vi "Snap Camera Image.vi"(7 "Test Recipe in":refnum<class "Test Recipe.lvclass">, 10 "Camera":refnum<class "Camera.lvclass">, 11 "Path":path) -> (0 "error out":errorcluster, 2 "No Artifacts Found":bool, 3 "LEDs Found":u32)   [LabVIEW 2015, in "LED Board Test.lvclass"]
uses:
  LED Board Test.lvclass
  Classes/Instruments/Camera/Camera/Class/Camera.lvclass
  Classes/Test Recipe/Class/Test Recipe.lvclass
  Classes/Instruments/Camera/Camera/Vision Algorithm/Count LEDS on Image/Count LEDs on Image.lvclass
  Classes/Instruments/Camera/Camera/Vision Algorithm/Find Color Artifacts/Find Color Artifacts.lvclass
  Classes/Instruments/Camera/Camera/Vision Algorithm/Find Color Artifacts/Find Color Artifacts.lvclass/Find Color Artifacts.ctl
  Classes/Instruments/Camera/Camera/Vision Algorithm/Count LEDS on Image/Count LEDs on Image.lvclass/Count LEDs on Image.ctl
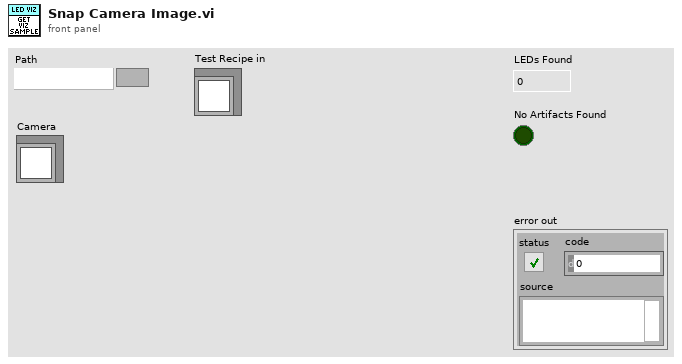
[diagram p1: front panel]
types:
  T1 = cluster{"Red Range":cluster{"Lower value":i32, "Upper value":i32}, "Green Range":cluster{"Lower value":i32, "Upper value":i32}, "Blue Range":cluster{"Lower value":i32, "Upper value":i32}}
  T2 = typedef "IMAQ Rectangle" = cluster{"Left":i32, "Top":i32, "Right":i32, "Bottom":i32, "Rotation":dbl}
  T3 = cluster{"Threshold":u32, "Min Size":u32, "Max Size":u32, "Use Max Size":bool}
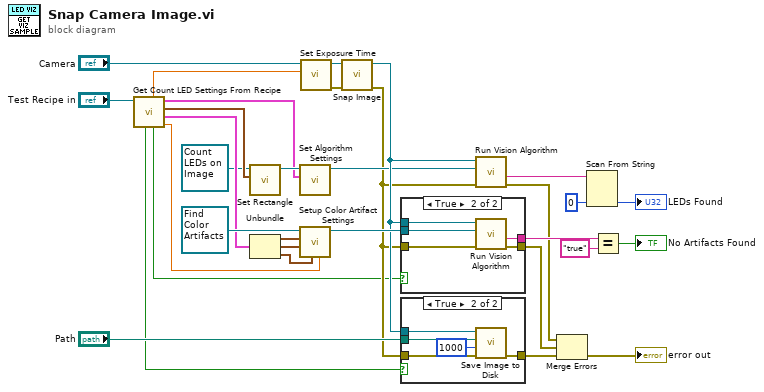
[diagram p0: block diagram]
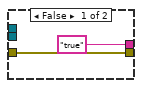
[diagram p2: hidden frame]
diagram:
  n1 = call "Get Count LED Settings From Recipe.vi"("Test Recipe in"="Test Recipe in") -> ("Minimum Artifact Size"=w3:dbl, "Threshold Values"=w23:T1, "Rectangle"=w26:T2, "Search Settings"=w10:T3, "Color?"=w1:bool, "Exposure Speed"=w13:dbl, "Save Image"=w2:bool)  [unwired: 4 in]
  n2 = call "Set Rectangle.vi"("Rectangle"=w26, "Count LEDs on Image in"=refnum<class "Count LEDs on Image.lvclass"> refnum ("Camera.lvlib:Count LEDs on Image.lvclass")) -> ("Count LEDs on Image out"=w12:refnum<class "Count LEDs on Image.lvclass">)  [unwired: 8 in, 1 out]
  n3 = Unbundle(w23) -> ("Red Range"=w22:cluster{"Lower value":i32, "Upper value":i32}, "Green Range"=w21:cluster{"Lower value":i32, "Upper value":i32}, "Blue Range"=w20:cluster{"Lower value":i32, "Upper value":i32})
  n4 = call "Set Algorithm Settings.vi"("Search Settings"=w10, "Count LEDs on Image in"=w12) -> ("Count LEDs on Image out"=w9:refnum<class "Count LEDs on Image.lvclass">)  [unwired: 8 in, 1 out]
  n5 = call "Setup Color Artifact Settings.vi"("Minimum Artifact Size"=w3, "Blue Range"=w20, "Green Range"=w21, "Red Range"=w22, "Find Color Artifacts in"=refnum<class "Find Color Artifacts.lvclass"> refnum ("Camera.lvlib:Find Color Artifacts.lvclass")) -> ("Find Color Artifacts out"=w19:refnum<class "Find Color Artifacts.lvclass">)  [unwired: 5 in, 1 out]
  n6 = call-dynamic "Set Exposure Time.vi"("Exposure Time"=w13, "Acrobat Template in"="Camera") -> ("error out"=w17:errorcluster, "Acrobat Template out"=w30:refnum<class "Camera.lvclass">)  [unwired: 8 in]
  n7 = call-dynamic "Snap Image.vi"("error in (no error)"=w17, "Acrobat Template in"=w30) -> ("error out"=w4:errorcluster, "Acrobat Template out"=w18:refnum<class "Camera.lvclass">)  [unwired: 8 in]
  n8 = case shown="True" w1 {
    tunnel: w19 -> [_ w39]
    tunnel: w18 -> [_ w38]
    tunnel: ["true" ("y") w37] -> w16
    tunnel: [w34 w36] -> w5
    tunnel: w4 -> [w34 w35]
    frame False {
    }
    frame True {
      n9 = call "Run Vision Algorithm.vi"("error in (no error)"=w35, "Vision Algorithm"=w39, "Camera in"=w38) -> ("error out"=w36:errorcluster, "Data"=w37:string)  [unwired: 4 in, 3 out]
    }
  }
  n10 = case shown="True" w2 {
    tunnel: "Path" -> [_ w45]
    tunnel: w18 -> [_ w44]
    tunnel: [w40 w43] -> w8
    tunnel: w4 -> [w40 w42]
    frame False {
    }
    frame True {
      n11 = call "Save Image to Disk.vi"("error in (no error)"=w42, "Image Quality (250)"=u32 1000, "Path"=w45, "Camera in"=w44) -> ("error out"=w43:errorcluster)  [unwired: 7 in]
    }
  }
  n12 = call "Run Vision Algorithm.vi"("error in (no error)"=w4, "Vision Algorithm"=w9, "Camera in"=w18) -> ("error out"=w6:errorcluster, "Data"=w25:string)  [unwired: 4 in, 3 out]
  n13 = Merge Errors(w6, w5, w8) -> (→"error out":errorcluster)
  n14 = Scan From String(input string=w25, default 1=0) -> (output 1=→"LEDs Found":i32)  [unwired: 3 in, 3 out]
  n15 = Equal?(x=w16, y="true") -> (x = y?=→"No Artifacts Found":bool)
